vi "PS90_PositionEx.vi"(5 "dValue-In":dbl format="%.4f", 6 "read?":bool, 7 "error in (no error)":errorcluster, 8 "Axis number":i32=1 min=1 max=9, 9 "Control unit ID":i32=1 min=1 max=10, 10 "DLOwis.lvclass":refnum<class "DLOwis.lvclass">) -> (0 "error out":errorcluster, 3 "DLOwis.lvclass":refnum<class "DLOwis.lvclass">, 4 "dValue-Out":dbl format="%.4f")   [LabVIEW 2020, in "DLOwis.lvclass"]
doc: "PS90_PositionEx.vi, created: 13.11.2006 alex; last change: 21.07.2016 alex;\n\n<B>FUNCTIONS:</B> \n\n<B>Read:</B> FALSE: read current value of a position counter \nof an axis (values in selected unit).\n<B>Write:</B> TRUE: set current value of a position counter\nof an axis (values in selected unit).\n----------------------------------------------------------------------------------------\n<B>INPUT:</B>\n[TF] <B>function:</B> function selector. (Read, Write)\n[I32] <B>Control unit ID:</B> control unit index. (Default=1, Range=1...10)\n[I32] <B>Axis number:</B> axis number. (Default=1, Range=1...9)\n[DBL] <B>dValue-In:</B> current position value. (only for Write: Default=0.0)\n[CLU] <B>error in</B>\n----------------------------------------------------------------------------------------\n<B>OUTPUT:</B>\n[DBL] <B>dValue-Out:</B> current position value. (for Write: dValue-Out=dValue-In)\n[CLU] <B>error out</B>\n----------------------------------------------------------------------------------------\n<B>SUB-VIs:</B>\nPS90_GetReadError.vi\n----------------------------------------------------------------------------------------\n<B>EXT-Calls:</B>\nps90.dll (V2.00)\n----------------------------------------------------------------------------------------"
uses:
  DLOwis.lvclass
  C:/dev/TRANCON/Classes/Delay Line/DelayLine.lvclass
  DelayLine.lvclass/DelayLine.ctl
  DelayLine.lvclass
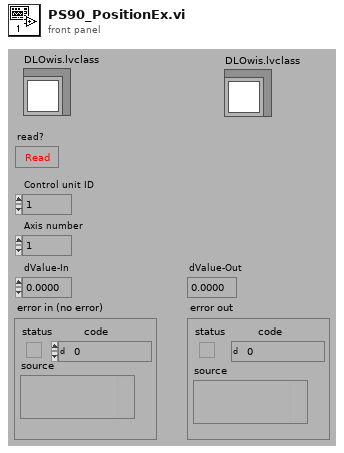
[diagram p1: front panel]
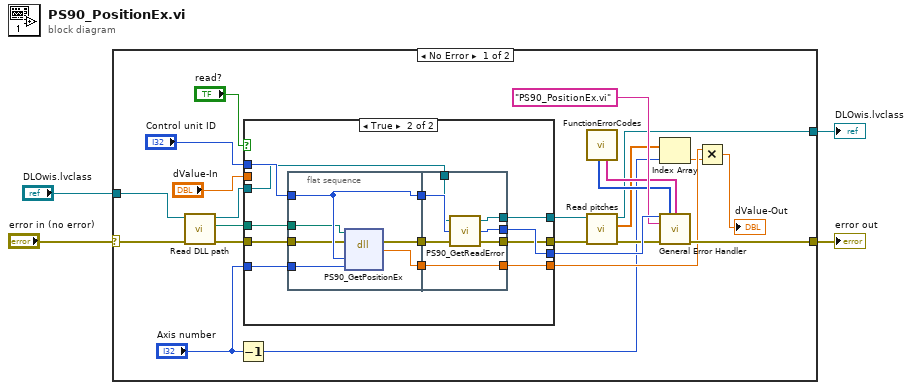
[diagram p0: block diagram]
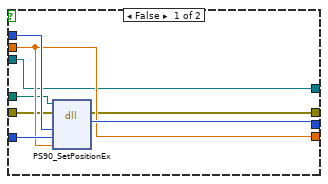
[diagram p2: hidden frame]
diagram:
  n1 = case shown="No Error" "error in (no error)" {
    selector: "error in (no error)" -> [w16 w61]
    tunnel: [w27 w61] -> w4
    tunnel: "DLOwis.lvclass" -> [w17 w62]
    tunnel: [w13 w62] -> w1
    frame No Error {
      n2 = call "Read DLL path.vi"("error in (no error)"=w16, "DelayLine in"=w17) -> ("error out"=w19:errorcluster, "DLL path"=w18:path, "DelayLine out"=w15:refnum<class "DLOwis.lvclass">)  [unwired: 7 in]
      n3 = Decrement(x="Axis number") -> (x-1=w5:i32)
      n4 = case shown="True" "read?" {
        tunnel: "Control unit ID" -> [w34 w46]
        tunnel: [w35 w47] -> w24
        tunnel: "dValue-In" -> [w32 _]
        tunnel: [w32 w45] -> w12
        tunnel: "Axis number" -> [w33 w44]
        tunnel: [w31 w40] -> w10
        tunnel: w19 -> [w29 w39]
        tunnel: w18 -> [w30 w38]
        tunnel: w15 -> [w28 w37]
        tunnel: [w28 w36] -> w14
        frame False {
          n5 = dll-call lib="C:/Users/Sergey Denisov/Documents/REPS/TRANCON/DLL/ps90.dll" fn="PS90_SetPositionEx" label="PS90_Set\nPositionEx"(path in=w30, error in=w29, "Index"=w34, "AxisNr"=w33, "dValue"=w32) -> (error out=w31:errorcluster, "Rückgabetyp"=w35:i32)  [unwired: 4 in, 1 out]
        }
        frame True {
          n6 = flat-sequence {
            tunnel: w46 -> [w53]
            tunnel: [w53] -> w43
            tunnel: [w52] -> w42
            tunnel: w44 -> [w51]
            tunnel: [w50] -> w41
            tunnel: w39 -> [w49]
            tunnel: w38 -> [w48]
            tunnel: [w60] -> w47
            tunnel: w43 -> [w59]
            tunnel: [w58] -> w45
            tunnel: w42 -> [w58]
            tunnel: w41 -> [w57]
            tunnel: [w56] -> w40
            tunnel: w37 -> [w55]
            tunnel: [w54] -> w36
            frame #0 {
              n7 = dll-call lib="C:/Users/Sergey Denisov/Documents/REPS/TRANCON/DLL/ps90.dll" fn="PS90_GetPositionEx" label="PS90_Get\nPositionEx"(path in=w48, error in=w49, "Index"=w53, "AxisNr"=w51) -> (error out=w50:errorcluster, "Rückgabetyp"=w52:dbl)  [unwired: 3 in, 1 out]
            }
            frame #1 {
              n8 = call "PS90_GetReadError.vi"("error in (no error)"=w57, "Control unit ID"=w59, "DLOwis.lvclass"=w55) -> ("error IO"=w56:errorcluster, "Read error"=w60:i32, "DLOwis.lvclass"=w54:refnum<class "DLOwis.lvclass">)
            }
          }
        }
      }
      n9 = call "FunctionErrorCodes.vi"() -> ("[user-defined codes]"=w21:i32[], "[user-defined descriptions]"=w20:string[])  [unwired: 8 in]
      n10 = call-dynamic "Read pitches.vi"("error in (no error)"=w10, "DelayLine in"=w14) -> ("error out"=w9:errorcluster, "pitches"=w7:dbl[], "DelayLine out"=w13:refnum<class "DLOwis.lvclass">)  [unwired: 7 in]
      n11 = Index Array(array=w7, index=w5) -> (element=w6:dbl)
      n12 = call <vilib>:"General Error Handler.vi"("[error code] (0)"=w24, "[user-defined codes]"=w21, "[user-defined descriptions]"=w20, "[error source] (\" \")"="PS90_PositionEx.vi" ("[error source] (\" \")"), "error in (no error)"=w9) -> ("error out"=w27:errorcluster)  [unwired: 6 in, 4 out]
      n13 = Multiply(x=w12, y=w6) -> (x*y=→"dValue-Out":dbl)
    }
    frame Error {
    }
  }
  "error out" <- w4
  "DLOwis.lvclass" <- w1
